vi "Max module time.vi"(10 "Module Array":T1(array[cluster])=[{"Enable"=TRUE, "Abs Start Time"=0.1, "Module"=0, "String"="dynamic DAC trigger", "Array"=["D", "14"]}, {"Enable"=TRUE, "Abs Start Time"=10.0, "Module"=1, "String"="trigger down", "Array"=["D", "14"]}, {"Enable"=TRUE, "Abs Start Time"=947.0, "Module"=19, "String"="", "Array"=[]}, {"Enable"=TRUE, "Abs Start Time"=947.0, "Module"=20, "String"="K trap freq for CMOT", "Array"=["5", "4.6"]}, {"Enable"=TRUE, "Abs Start Time"=947.0, "Module"=20, "String"="E/W shim for Qtrap loading", "Array"=["0", "-1"]}, {"Enable"=TRUE, "Abs Start Time"=947.0, "Module"=20, "String"="U/D shim for Qtrap loading", "Array"=["1", "-1.5"]}, {"Enable"=TRUE, "Abs Start Time"=947.0, "Module"=20, "String"="N/S shim for Qtrap loading", "Array"=["2", "-1"]}, {"Enable"=TRUE, "Abs Start Time"=947.0, "Module"=20, "String"="repump K freq for OP", "Array"=["3", "0.05"]}, {"Enable"=TRUE, "Abs Start Time"=994.5, "Module"=20, "String"="E/W shim for molasses 0", "Array"=["0", "-1"]}, {"Enable"=TRUE, "Abs Start Time"=994.5, "Module"=20, "String"="U/D shim for molasses -0.6", "Array"=["1", "0.1"]}, {"Enable"=TRUE, "Abs Start Time"=994.5, "Module"=20, "String"="N/S shim for molasses 0", "Array"=["2", "2"]}, {"Enable"=TRUE, "Abs Start Time"=995.5, "Module"=8, "String"="", "Array"=["", ""]}, {"Enable"=TRUE, "Abs Start Time"=997.1, "Module"=1, "String"="close Rb shutter(takes 1.4 ms", "Array"=["B", "0"]}, {"Enable"=FALSE, "Abs Start Time"=998.5, "Module"=12, "String"="\n", "Array"=[]}, {"Enable"=FALSE, "Abs Start Time"=998.5, "Module"=0, "String"="scope trigger", "Array"=["c", "7"]}, {"Enable"=FALSE, "Abs Start Time"=999.0, "Module"=1, "String"="", "Array"=["c", "7"]}, {"Enable"=TRUE, "Abs Start Time"=1000.0, "Module"=14, "String"="", "Array"=[]}, {"Enable"=TRUE, "Abs Start Time"=1000.0, "Module"=20, "String"="K trap freq for MOT", "Array"=["5", "4.3"]}, {"Enable"=TRUE, "Abs Start Time"=1000.0, "Module"=20, "String"=" K repump freq for MOT freq", "Array"=["3", "0"]}, {"Enable"=TRUE, "Abs Start Time"=1000.0, "Module"=20, "String"="E/W shim for Qtrap", "Array"=["0", "2"]}, {"Enable"=TRUE, "Abs Start Time"=1000.0, "Module"=20, "String"="U/D shim for Qtrap", "Array"=["1", "2"]}, {"Enable"=TRUE, "Abs Start Time"=1000.0, "Module"=20, "String"="N/S shim for Qtrap", "Array"=["2", "2"]}, {"Enable"=TRUE, "Abs Start Time"=1000.0, "Module"=10, "String"="", "Array"=["-10"]}, {"Enable"=TRUE, "Abs Start Time"=1000.0, "Module"=0, "String"="laser unlock", "Array"=["A", "1"]}, {"Enable"=TRUE, "Abs Start Time"=2400.0, "Module"=1, "String"="laser relock", "Array"=["A", "1"]}, {"Enable"=FALSE, "Abs Start Time"=2900.0, "Module"=0, "String"="", "Array"=["c", "7"]}, {"Enable"=TRUE, "Abs Start Time"=2900.0, "Module"=8, "String"="", "Array"=[]}, {"Enable"=TRUE, "Abs Start Time"=2800.0, "Module"=0, "String"="IP bias bleed on", "Array"=["B", "3"]}, {"Enable"=TRUE, "Abs Start Time"=2900.0, "Module"=0, "String"="IP master switch on", "Array"=["B", "2"]}, {"Enable"=FALSE, "Abs Start Time"=2905.0, "Module"=11, "String"="", "Array"=[]}, {"Enable"=FALSE, "Abs Start Time"=4400.0, "Module"=0, "String"="laser unlock for return", "Array"=["A", "1"]}, {"Enable"=FALSE, "Abs Start Time"=5900.0, "Module"=1, "String"="laser unlock for return", "Array"=["A", "1"]}, {"Enable"=FALSE, "Abs Start Time"=6000.0, "Module"=20, "String"="E/W shim for MOT", "Array"=["0", "0"]}, {"Enable"=FALSE, "Abs Start Time"=6000.0, "Module"=20, "String"="U/D shim for MOT", "Array"=["1", "-1"]}, {"Enable"=FALSE, "Abs Start Time"=6000.0, "Module"=20, "String"="N/S shim for MOT", "Array"=["2", "-1.5"]}, {"Enable"=FALSE, "Abs Start Time"=20900.0, "Module"=3, "String"="", "Array"=[]}, {"Enable"=FALSE, "Abs Start Time"=11035.078497322447, "Module"=0, "String"="", "Array"=[]}, {"Enable"=TRUE, "Abs Start Time"=14135.078497322447, "Module"=1, "String"="IP master switch off", "Array"=["B", "2"]}, {"Enable"=TRUE, "Abs Start Time"=14135.078497322447, "Module"=0, "String"="trigger scope", "Array"=["c", "7"]}, {"Enable"=TRUE, "Abs Start Time"=14140.078497322447, "Module"=11, "String"="", "Array"=[]}, {"Enable"=TRUE, "Abs Start Time"=15635.078497322447, "Module"=0, "String"="laser unlock for cart return", "Array"=["A", "1"]}, {"Enable"=TRUE, "Abs Start Time"=17135.078497322447, "Module"=1, "String"="laser relock", "Array"=["A", "1"]}, {"Enable"=TRUE, "Abs Start Time"=17135.078497322447, "Module"=20, "String"="E/W shim for MOT", "Array"=["0", "0"]}, {"Enable"=TRUE, "Abs Start Time"=17135.078497322447, "Module"=20, "String"="U/D shim for MOT", "Array"=["1", "-1"]}, {"Enable"=TRUE, "Abs Start Time"=17135.078497322447, "Module"=20, "String"="N/S shim for MOT", "Array"=["2", "-1.5"]}, {"Enable"=TRUE, "Abs Start Time"=17235.078497322447, "Module"=3, "String"="", "Array"=[]}, {"Enable"=FALSE, "Abs Start Time"=32135.078497322447, "Module"=3, "String"="", "Array"=[]}, {"Enable"=TRUE, "Abs Start Time"=15135.078497322447, "Module"=0, "String"="", "Array"=["c", "7"]}, {"Enable"=TRUE, "Abs Start Time"=17335.078497322447, "Module"=1, "String"="", "Array"=["c", "7"]}] {"Abs Start Time" format="%.2f"}) -> (2 "max value":dbl)   [LabVIEW 2017]
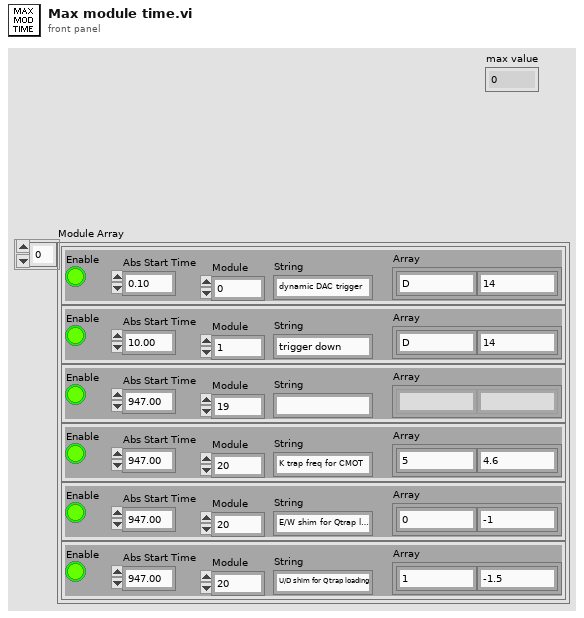
[diagram p1: front panel]
types:
  T1 = cluster{"Enable":bool, "Abs Start Time":dbl, "Module":u16, "String":string, "Array":string[]}[]
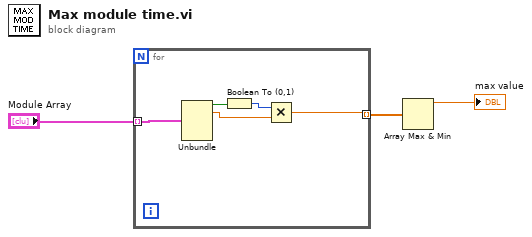
[diagram p0: block diagram]
diagram:
  n1 = for {
    tunnel: "Module Array" -> [w8] mode=indexing
    tunnel: [w4] -> w2 mode=indexing
    n2 = Unbundle(w8) -> ("Enable"=w7:bool, "Abs Start Time"=w5:dbl)  [unwired: 3 out]
    n3 = Boolean To (0,1)(Boolean=w7) -> (0, 1=w6:i16)
    n4 = Multiply(x=w6, y=w5) -> (x*y=w4:dbl)
  }
  n5 = Array Max & Min(array=w2) -> (max value=→"max value":dbl)  [unwired: 3 out]
